vi "序号表头生成.vi"(8 "error in (no error)":errorcluster caption="错误输入（无错误）", 10 "替换起始列":bool=TRUE, 11 "表格数据":string[][](array[string])) -> (0 "error out":errorcluster caption="错误输出", 3 "输出数组":string[][](array[string]))   [LabVIEW 2014, in "表格.lvlib"]
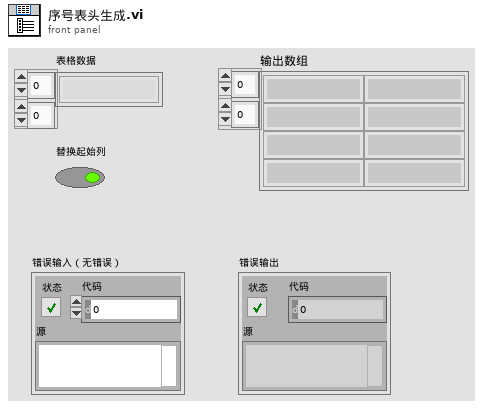
[diagram p1: front panel]
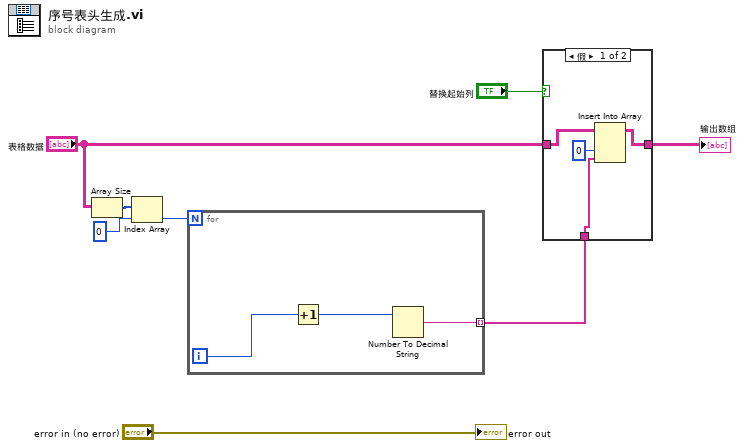
[diagram p0: block diagram]
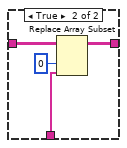
[diagram p2: hidden frame]
diagram:
  n1 = Array Size(array="表格数据") -> (size(s)=w8:i32[])
  n2 = Index Array(array=w8, index=0 ("索引")) -> (element=w6:i32)
  n3 = for {
    N: w6 -> [_]
    tunnel: [w9] -> w4 mode=indexing
    i -> [w11]
    n4 = Increment(x=w11) -> (x+1=w10:i32)
    n5 = Number To Decimal String(number=w10) -> (decimal integer string=w9:string)  [unwired: 1 in]
  }
  n6 = case shown="假" "替换起始列" {
    tunnel: "表格数据" -> [w15 w19]
    tunnel: w4 -> [w13 w18]
    tunnel: [w12 w16] -> w3
    frame False {
      n7 = Insert Into Array(array=w15, index (col)=0 ("禁用的索引 (列)"), new element=w13) -> (w12:string[][])  [unwired: 1 in]
    }
    frame True {
      n8 = Replace Array Subset(array=w19, new element=w18, index (col)=0 ("禁用的索引 (列)")) -> (w16:string[][])  [unwired: 1 in]
    }
  }
  "输出数组" <- w3
  "error out" <- "error in (no error)"
